vi "SaveState.vi"() -> ()   [LabVIEW 2017]
uses:
  TestControl.ctl
panel:
  in  "Cluster":T1
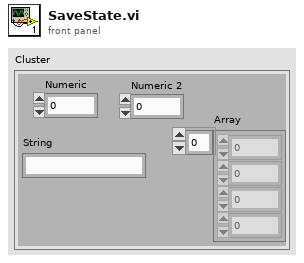
[diagram p1: front panel]
types:
  T1 = typedef "TestControl.ctl" = cluster{"Array":dbl[], "String":string, "Numeric":dbl, "Numeric 2":dbl}
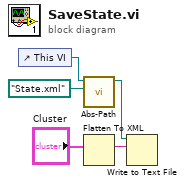
[diagram p0: block diagram]
diagram:
  n1 = control-ref of="This VI"() -> (w3:refnum<vi>)
  n2 = call "Abs-Path.vi"("filename"=path "State.xml" ("file (use dialog)"), "Vi in path"=w3) -> ("Full path"=w1:path)  [unwired: 9 in]
  n3 = Flatten To XML(anything="Cluster") -> (xml string=w5:string)
  n4 = Write to Text File(file (use dialog)=w1, text=w5) -> ()  [unwired: 2 in, 3 out]
